vi "Wait for Data Acquisition Complete.vi"(8 "error in (no error)":errorcluster, 10 "Maximum Time (10000 ms)":u32=10000, 11 "VISA resource name":refnum<visa-resource-name>) -> (0 "error out":errorcluster, 3 "VISA resource name out":refnum<visa-resource-name>)   [LabVIEW 2020, in "Library Instrument & Equipement.lvlib" / "Library Multimeter.lvlib" / "RIGOL DM3058.lvlib"]
doc: "Waits for the data acquisition operation complete.\n\n<B>Note:</B>\nThis VI only applies for RIGOL DM3051 model with firmware 03.12.00.03.04.00.07 or later."
uses:
  RIGOL DM3058.lvlib
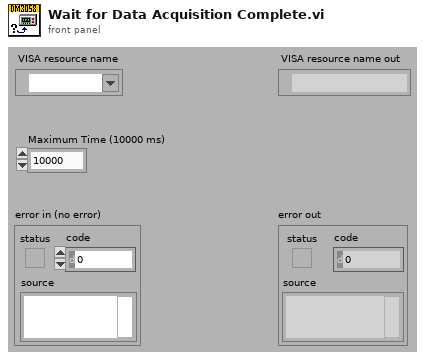
[diagram p1: front panel]
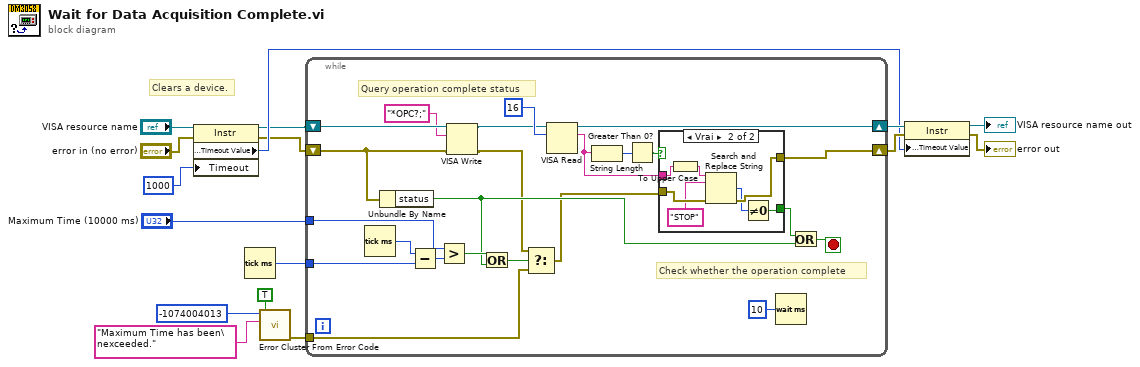
[diagram p0: block diagram]
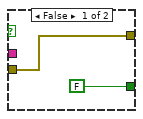
[diagram p2: hidden frame]
diagram:
  # "Clears a device."
  n1 = property class="Instr"(reference="VISA resource name", error in="error in (no error)", "Timeout"=u32 1000 ("General Settings:Timeout Value")) -> (reference out=w2:refnum<visa-resource-name>, error out=w1:errorcluster, "General Settings:Timeout Value"=w4:u32)
  n2 = Tick Count (ms)() -> (millisecond timer value=w16:u32)
  n3 = call <vilib>:"Error Cluster From Error Code.vi"("show call chain? (False)"=TRUE, "error message (\"\")"="Maximum Time has been\nexceeded." ("error message (\"\")"), "error code (0)"=-1074004013) -> ("error out"=w12:errorcluster)  [unwired: 1 in, 5 out]
  n4 = while {
    tunnel: "Maximum Time (10000 ms)" -> [w33]
    tunnel: w16 -> [w36]
    tunnel: w12 -> [w28]
    shift-right: [w35] -> w6
    shift-left: w1 -> [w18]
    shift-right: [w39] -> w8
    shift-left: w2 -> [w19]
    stop <- w34 stop-if-true
    # "Query operation complete status"
    # "Check whether the operation complete"
    n5 = Tick Count (ms)() -> (millisecond timer value=w37:u32)
    n6 = Unbundle By Name(w18) -> ("status"=w29:bool)
    n7 = Subtract(x=w37, y=w36) -> (x-y=w32:u32)
    n8 = Greater?(x=w33, y=w32) -> (0:w31:bool)
    n9 = VISA Write(VISA resource name=w19, write buffer="*OPC?;", error in (no error)=w18) -> (VISA resource name out=w21:refnum<visa-resource-name>, error out=w20:errorcluster)  [unwired: 1 out]
    n10 = Or(x=w31, y=w29) -> (x .or. y?=w30:bool)
    n11 = Select(t=w20, s=w30, f=w28) -> (s? t:f=w25:errorcluster)
    n12 = VISA Read(VISA resource name=w21, byte count=u32 16) -> (VISA resource name out=w39:refnum<visa-resource-name>, read buffer=w22:string)  [unwired: 1 in, 2 out]
    n13 = String Length(string=w22) -> (length=w24:i32)
    n14 = Greater Than 0?(x=w24) -> (x > 0?=w23:bool)
    n15 = case shown="Vrai" w23 {
      tunnel: [w41 w45] -> w35
      tunnel: [FALSE w43] -> w26
      tunnel: w25 -> [w41 w46]
      tunnel: w22 -> [_ w48]
      frame False {
      }
      frame True {
        n16 = To Upper Case(1:w48) -> (0:w47:string)
        n17 = Search and Replace String(input string=w47, search string="STOP" ("y"), error in=w46) -> (number of replacements=w42:i32, error out=w45:errorcluster)  [unwired: 7 out]
        n18 = Not Equal To 0?(x=w42) -> (x != 0?=w43:bool)
      }
    }
    n19 = Wait (ms)(milliseconds to wait=u32 10) -> ()  [unwired: 1 out]
    n20 = Or(x=w26, y=w29) -> (x .or. y?=w34:bool)
  }
  n21 = property class="Instr"(reference=w8, error in=w6, "General Settings:Timeout Value"=w4) -> (reference out=→"VISA resource name out":refnum<visa-resource-name>, error out=→"error out":errorcluster)
